vi "S4_Youngs_Graph.vi"() -> ()   [LabVIEW 2012]
uses:
  2015myGlobal 1.vi
  <vilib>/Utility/file.llb/Write To Spreadsheet File (DBL).vi
panel:
  in  "Tab Control":enum32{"Chart", "X-Y Plot"}(tab)
  out "Chart of  Fource & Dislpacement":cluster{"步進馬達位置":i32, "Fource_LoadCell (V)":dbl}(graph)
  out "XY Graph":cluster{i32[], dbl[]}(graph)
  in  "stop":bool
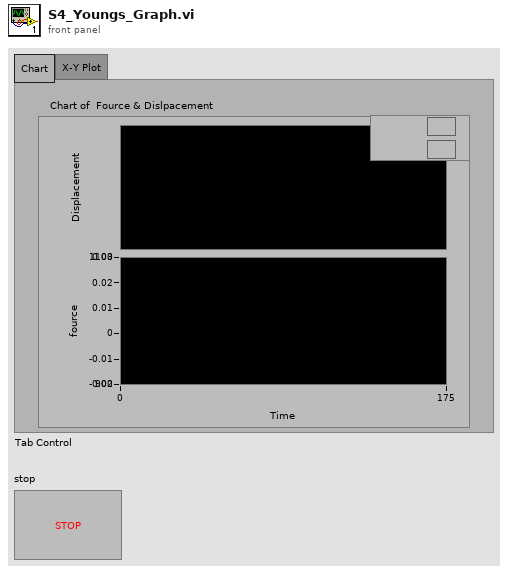
[diagram p1: front panel]
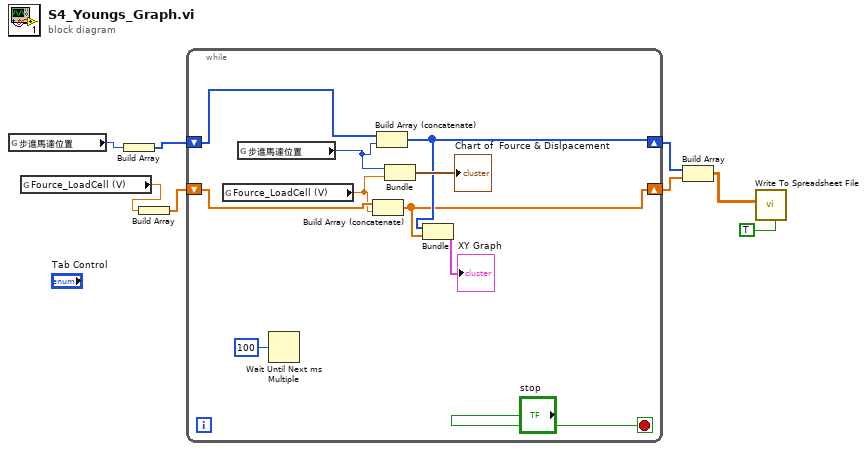
[diagram p0: block diagram]
diagram:
  n1 = global read "2015myGlobal 1.vi" "步進馬達位置"() -> (w8:i32)
  n2 = global read "2015myGlobal 1.vi" "Fource_LoadCell (V)"() -> (w6:dbl)
  n3 = Build Array(w8) -> (w7:i32[])
  n4 = Build Array(w6) -> (w5:dbl[])
  n5 = while {
    shift-right: [w11] -> w4
    shift-left: w7 -> [w15]
    shift-right: [w10] -> w3
    shift-left: w5 -> [w13]
    stop <- "stop" stop-if-true
    n6 = global read "2015myGlobal 1.vi" "Fource_LoadCell (V)"() -> (w12:dbl)
    n7 = global read "2015myGlobal 1.vi" "步進馬達位置"() -> (w14:i32)
    n8 = Wait Until Next ms Multiple(millisecond multiple=u32 100) -> ()  [unwired: 1 out]
    n9 = Build Array (concatenate)(w13, w12) -> (w10:dbl[])
    n10 = Build Array (concatenate)(w15, w14) -> (w11:i32[])
    n11 = Bundle("步進馬達位置"=w14, "Fource_LoadCell (V)"=w12) -> (→"Chart of  Fource & Dislpacement":cluster{"步進馬達位置":i32, "Fource_LoadCell (V)":dbl})  [unwired: 1 in]
    n12 = Bundle(w11, w10) -> (→"XY Graph":cluster{i32[], dbl[]})  [unwired: 1 in]
  }
  n13 = Build Array(w4, w3) -> (w2:dbl[][])
  n14 = call-poly <vilib>:"Write To Spreadsheet File.vi"("transpose? (no:F)"=TRUE, "2D data"=w2) -> ()  [unwired: 6 in, 1 out]
